vi "Correct-sign.vi"(8 "error in (no error)":errorcluster, 10 "Value in":dbl caption="Value in [unit]", 11 "Motor in":refnum<class "Motor.lvclass">) -> (0 "error out":errorcluster, 2 "Value out":dbl, 3 "Motor out":refnum<class "Motor.lvclass">)   [LabVIEW 2013, in "PowderDeposition.lvlib" / "Motor.lvclass"]
uses:
  Motor.lvclass
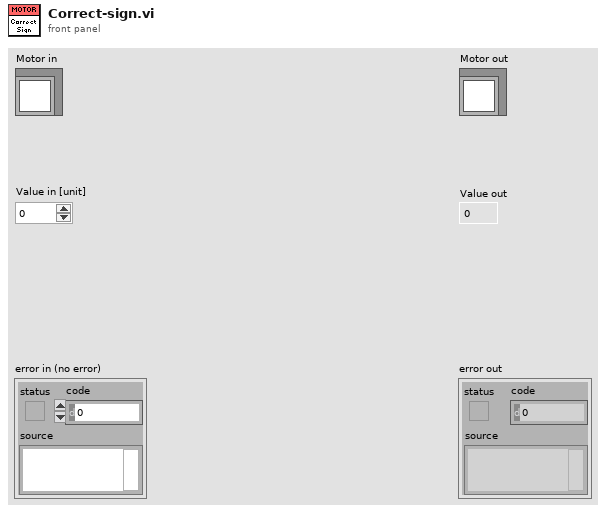
[diagram p1: front panel]
types:
  T1 = typedef "Action-settings.ctl" = cluster{"Speed":dbl, "Acceleration":dbl, "Direction":enum16{"Clockwise", "Counter-clockwise"}}
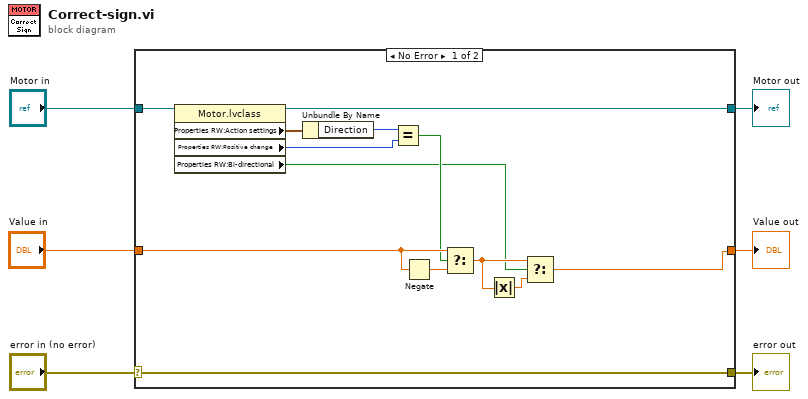
[diagram p0: block diagram]
diagram:
  n1 = case shown="No Error" "error in (no error)" {
    selector: "error in (no error)" -> [w18 w22]
    tunnel: [w18 w22] -> w5
    tunnel: [w17 w21] -> w3
    tunnel: "Motor in" -> [w19 w21]
    tunnel: "Value in" -> [w12 w20]
    tunnel: [w7 w20] -> w1
    frame No Error {
      n2 = property class="Motor.lvclass"(reference=w19) -> (reference out=w17:refnum<class "Motor.lvclass">, "Properties RW:Action settings"=w16:T1, "Properties RW:Positive change"=w14:enum16{"Clockwise", "Counter-clockwise"}, "Properties RW:Bi-directional"=w8:bool)  [unwired: 1 in, 1 out]
      n3 = Unbundle By Name(w16) -> ("Direction"=w15:enum16{"Clockwise", "Counter-clockwise"})
      n4 = Equal?(x=w15, y=w14) -> (x = y?=w11:bool)
      n5 = Negate(x=w12) -> (-x=w13:dbl)
      n6 = Select(t=w12, s=w11, f=w13) -> (s? t:f=w9:dbl)
      n7 = Absolute Value(x=w9) -> (abs(x)=w10:dbl)
      n8 = Select(t=w9, s=w8, f=w10) -> (s? t:f=w7:dbl)
    }
    frame Error {
    }
  }
  "error out" <- w5
  "Motor out" <- w3
  "Value out" <- w1
